vi "String Array to String with Commas.vi"(1 "Array":string[](array[string])) -> (0 "String":string)   [LabVIEW 2013, in "Data.PGSQL.lvclass"]
uses:
  Data.PGSQL.lvclass
panel:
  out "should it be this?":string
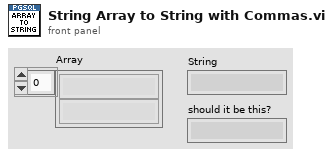
[diagram p1: front panel]
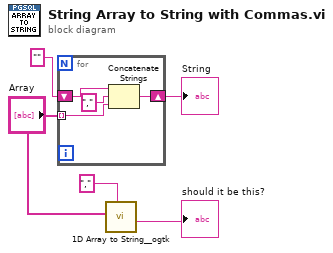
[diagram p0: block diagram]
diagram:
  n1 = for {
    tunnel: "Array" -> [w6] mode=indexing
    shift-right: [w9] -> w4
    shift-left: "" -> [w8]
    n2 = Concatenate Strings(w8, "," ("string"), w6) -> (w9:string)
  }
  "String" <- w4
  n3 = call "1D Array to String__ogtk.vi"("delimiter (Tab)"="," ("string"), "Array of Strings"="Array") -> ("delimited string"=→"should it be this?":string)  [unwired: 9 in]
